vi "输入数据解析.vi"(0 "单个参数补充":dbl, 1 "从板号":dbl=1.0, 2 "主板二维码":string="BNET01", 3 "从板二维码":string="BNET01", 5 "主板引用":refnum<vi>, 7 "从板引用":refnum<vi>, 9 "主板选项":string="三级故障阀值", 11 "枚举":enum16{"主板", "从板"}(ring), 12 "快换":bool caption="快换写入") -> (4 "输出数组":dbl[][](array[numeric]), 6 "数组长度":dbl[](array[numeric]), 8 "循环次数":i32, 10 "命令":u32, 14 "名称":string[](array[string]), 15 "命令序号":u32[](array[numeric]))   [LabVIEW 2013] (continued)
                    n1944 = Unbundle By Name(w4966) -> ("总电压过低"=w4965:dbl)
                    n1945 = call "输入分辨率计算-EV05.vi"("1字节?"=FALSE, "数值"=w4965, "分辨率"=0.1) -> ("低字节"=w4968:dbl, "高字节1"=w4967:dbl)  [unwired: 2 in, 5 out]
                  }
                  frame Enabled {
                    w4971 = 255 ("高字节1")
                  }
                }
                n1946 = Build Array(w4963, w4964) -> (w4962:i32[])
              }
              frame 2 {
                # "温度过高"
                n1947 = disable-structure shown="启用" {
                  disable-tunnel: [w4978 255 ("高字节1")] -> w4974
                  disable-tunnel: w4972 -> [w4976 _]
                  frame Disabled {
                    n1948 = Unbundle By Name(w4976) -> ("温度过高"=w4975:dbl)
                    n1949 = call "输入分辨率计算-EV05.vi"("1字节?"=TRUE, "数值"=w4975, "偏移量"=-40.0, "分辨率"=1.0) -> ("高字节1"=w4978:dbl)  [unwired: 1 in, 6 out]
                  }
                  frame Enabled {
                  }
                }
                n1950 = Build Array(w4974) -> (w4973:i32[])
              }
              frame 3 {
                # "温度过低"
                n1951 = disable-structure shown="启用" {
                  disable-tunnel: [w4988 255 ("高字节1")] -> w4984
                  disable-tunnel: w4982 -> [w4986 _]
                  frame Disabled {
                    n1952 = Unbundle By Name(w4986) -> ("温度过低"=w4985:dbl)
                    n1953 = call "输入分辨率计算-EV05.vi"("1字节?"=TRUE, "数值"=w4985, "偏移量"=-40.0, "分辨率"=1.0) -> ("高字节1"=w4988:dbl)  [unwired: 1 in, 6 out]
                  }
                  frame Enabled {
                  }
                }
                n1954 = Build Array(w4984) -> (w4983:i32[])
              }
              frame 4 {
                # "整组温度不均衡"
                n1955 = disable-structure shown="启用" {
                  disable-tunnel: [w4998 255 ("高字节1")] -> w4994
                  disable-tunnel: w4992 -> [w4996 _]
                  frame Disabled {
                    n1956 = Unbundle By Name(w4996) -> ("整组温度不均衡"=w4995:dbl)
                    n1957 = call "输入分辨率计算-EV05.vi"("1字节?"=TRUE, "数值"=w4995, "偏移量"=0.0, "分辨率"=1.0) -> ("高字节1"=w4998:dbl)  [unwired: 1 in, 6 out]
                  }
                  frame Enabled {
                  }
                }
                n1958 = Build Array(w4994) -> (w4993:i32[])
              }
              frame 5 {
                # "单组电压不均衡"
                n1959 = disable-structure shown="启用" {
                  disable-tunnel: [w5010 w5013] -> w5005
                  disable-tunnel: [w5008 w5013] -> w5003
                  disable-tunnel: w5002 -> [w5007 _]
                  frame Enabled {
                    n1960 = Unbundle By Name(w5007) -> ("单组电压不均衡"=w5006:dbl)
                    n1961 = call "输入分辨率计算-EV05.vi"("1字节?"=FALSE, "数值"=w5006, "偏移量"=0.0, "分辨率"=0.001) -> ("低字节"=w5008:dbl, "高字节1"=w5010:dbl)  [unwired: 1 in, 5 out]
                  }
                  frame Disabled {
                    w5013 = 255 ("高字节1")
                  }
                }
                n1962 = Build Array(w5005, w5003) -> (w5004:dbl[])
              }
              frame 6 {
                # "整组电压不均衡"
                n1963 = disable-structure shown="启用" {
                  disable-tunnel: [w5022 w5025] -> w5017
                  disable-tunnel: [w5020 w5025] -> w5015
                  disable-tunnel: w5014 -> [w5019 _]
                  frame Disabled {
                    n1964 = Unbundle By Name(w5019) -> ("整组电压不均衡"=w5018:dbl)
                    n1965 = call "输入分辨率计算-EV05.vi"("1字节?"=FALSE, "数值"=w5018, "偏移量"=0.0, "分辨率"=0.001) -> ("低字节"=w5020:dbl, "高字节1"=w5022:dbl)  [unwired: 1 in, 5 out]
                  }
                  frame Enabled {
                    w5025 = 255 ("高字节1")
                  }
                }
                n1966 = Build Array(w5017, w5015) -> (w5016:i32[])
              }
              frame 7 {
                # "单体电压过高"
                n1967 = disable-structure shown="启用" {
                  disable-tunnel: [w5034 w5037] -> w5029
                  disable-tunnel: [w5032 w5037] -> w5027
                  disable-tunnel: w5026 -> [w5031 _]
                  frame Disabled {
                    n1968 = Unbundle By Name(w5031) -> ("单体电压过高"=w5030:dbl)
                    n1969 = call "输入分辨率计算-EV05.vi"("1字节?"=FALSE, "数值"=w5030, "偏移量"=0.0, "分辨率"=0.001) -> ("低字节"=w5032:dbl, "高字节1"=w5034:dbl)  [unwired: 1 in, 5 out]
                  }
                  frame Enabled {
                    w5037 = 255 ("高字节1")
                  }
                }
                n1970 = Build Array(w5029, w5027) -> (w5028:i32[])
              }
              frame 8 {
                # "单体电压过低"
                n1971 = disable-structure shown="启用" {
                  disable-tunnel: [w5046 w5049] -> w5041
                  disable-tunnel: [w5044 w5049] -> w5039
                  disable-tunnel: w5038 -> [w5043 _]
                  frame Disabled {
                    n1972 = Unbundle By Name(w5043) -> ("单体电压过低"=w5042:dbl)
                    n1973 = call "输入分辨率计算-EV05.vi"("1字节?"=FALSE, "数值"=w5042, "偏移量"=0.0, "分辨率"=0.001) -> ("低字节"=w5044:dbl, "高字节1"=w5046:dbl)  [unwired: 1 in, 5 out]
                  }
                  frame Enabled {
                    w5049 = 255 ("高字节1")
                  }
                }
                n1974 = Build Array(w5041, w5039) -> (w5040:i32[])
              }
              frame 9 {
                # "充电电流过高"
                n1975 = disable-structure shown="启用" {
                  disable-tunnel: [w5058 w5061] -> w5053
                  disable-tunnel: [w5056 w5061] -> w5051
                  disable-tunnel: w5050 -> [w5055 _]
                  frame Disabled {
                    n1976 = Unbundle By Name(w5055) -> ("充电电流过高"=w5054:dbl)
                    n1977 = call "输入分辨率计算-EV05.vi"("1字节?"=FALSE, "数值"=w5054, "偏移量"=-3000.0, "分辨率"=0.1) -> ("低字节"=w5056:dbl, "高字节1"=w5058:dbl)  [unwired: 1 in, 5 out]
                  }
                  frame Enabled {
                    w5061 = 255 ("高字节1")
                  }
                }
                n1978 = Build Array(w5053, w5051) -> (w5052:i32[])
              }
              frame 10 {
                # "放电电流过高"
                n1979 = disable-structure shown="启用" {
                  disable-tunnel: [w5070 w5073] -> w5065
                  disable-tunnel: [w5068 w5073] -> w5063
                  disable-tunnel: w5062 -> [w5067 _]
                  frame Disabled {
                    n1980 = Unbundle By Name(w5067) -> ("放电电流过高"=w5066:dbl)
                    n1981 = call "输入分辨率计算-EV05.vi"("1字节?"=FALSE, "数值"=w5066, "偏移量"=-3000.0, "分辨率"=0.1) -> ("低字节"=w5068:dbl, "高字节1"=w5070:dbl)  [unwired: 1 in, 5 out]
                  }
                  frame Enabled {
                    w5073 = 255 ("高字节1")
                  }
                }
                n1982 = Build Array(w5065, w5063) -> (w5064:i32[])
              }
              frame 11 {
                # "单组温度不均衡"
                n1983 = disable-structure shown="启用" {
                  disable-tunnel: [w5080 255 ("高字节1")] -> w5076
                  disable-tunnel: w5074 -> [w5078 _]
                  frame Disabled {
                    n1984 = Unbundle By Name(w5078) -> ("单组温度不均衡"=w5077:dbl)
                    n1985 = call "输入分辨率计算-EV05.vi"("1字节?"=TRUE, "数值"=w5077, "偏移量"=0.0, "分辨率"=1.0) -> ("高字节1"=w5080:dbl)  [unwired: 1 in, 6 out]
                  }
                  frame Enabled {
                  }
                }
                n1986 = Build Array(w5076) -> (w5075:i32[])
              }
              frame 12 {
                # "SOC过高"
                n1987 = Unbundle By Name(w5088) -> ("SOC过高"=w5087:dbl)
                n1988 = call "输入分辨率计算-EV05.vi"("1字节?"=FALSE, "数值"=w5087, "偏移量"=0.0, "分辨率"=0.1) -> ("低字节"=w5089:dbl, "高字节1"=w5090:dbl)  [unwired: 1 in, 5 out]
                n1989 = call "二进制解析-8.6.vi"("索引"=4, "数值"=w5090) -> ("低位子数组"=w5093:i32[])  [unwired: 3 out]
                n1990 = call "二进制解析-8.6.vi"("索引"=4, "数值"=w5089) -> ("低位子数组"=w5085:i32[], "高位子数组"=w5092:i32[])  [unwired: 2 out]
                n1991 = Insert Into Array(array=w5093, new element=w5092) -> (w5091:i32[])  [unwired: 1 in]
                n1992 = call "数值二进制转十进制-8.6.vi"("子数组"=w5091) -> ("十进制数值"=w5086:i32)  [unwired: 4 out]
                n1993 = disable-structure shown="启用" {
                  disable-tunnel: w5086 -> [w5101 _]
                  disable-tunnel: [w5101 255 ("高字节1")] -> w5084
                  disable-tunnel: [w5100 i32[] [] ("低位子数组 23")] -> _
                  disable-tunnel: w5085 -> [w5100 _]
                  frame Disabled {
                  }
                  frame Enabled {
                  }
                }
                n1994 = Build Array(w5084, w5084) -> (w5097:i32[])
              }
              frame 13 {
                # "SOC过低"
                n1995 = Unbundle By Name(w5110) -> ("SOC过低"=w5109:dbl)
                n1996 = call "输入分辨率计算-EV05.vi"("1字节?"=FALSE, "数值"=w5109, "偏移量"=0.0, "分辨率"=0.1) -> ("低字节"=w5107:dbl, "高字节1"=w5108:dbl)  [unwired: 1 in, 5 out]
                n1997 = call "二进制解析-8.6.vi"("索引"=4, "数值"=w5108) -> ("低位子数组"=w5105:i32[])  [unwired: 3 out]
                n1998 = disable-structure shown="启用" {
                  disable-tunnel: w5107 -> [w5117 _]
                  disable-tunnel: [w5117 255 ("高字节1")] -> w5106
                  disable-tunnel: w5105 -> [w5116 _]
                  disable-tunnel: [_ 255 ("高字节1")] -> w5104
                  frame Disabled {
                    (unwired) i32[] [] ("低位子数组 4")
                  }
                  frame Enabled {
                  }
                }
                n1999 = Build Array(w5104, w5106) -> (w5113:i32[])
              }
              frame 14 {
                # "内阻过大"
                n2000 = disable-structure shown="启用" {
                  disable-tunnel: w5122 -> [w5127 _]
                  disable-tunnel: [w5123 255 ("高字节1")] -> w5120
                  frame Disabled {
                    n2001 = Unbundle By Name(w5127) -> ("内阻过大"=w5126:dbl)
                    n2002 = call "输入分辨率计算-EV05.vi"("1字节?"=TRUE, "数值"=w5126, "分辨率"=0.1) -> ("高字节1"=w5123:dbl)  [unwired: 2 in, 6 out]
                  }
                  frame Enabled {
                  }
                }
                n2003 = Build Array(w5120) -> (w5121:i32[])
              }
              frame 15 {
                # "极柱温度过高"
                n2004 = disable-structure shown="启用" {
                  disable-tunnel: w5131 -> [w5137 _]
                  disable-tunnel: [w5133 255 ("高字节1")] -> w5129
                  frame Disabled {
                    n2005 = Unbundle By Name(w5137) -> ("极柱温度过高"=w5136:dbl)
                    n2006 = call "输入分辨率计算-EV05.vi"("1字节?"=TRUE, "数值"=w5136, "偏移量"=-40.0, "分辨率"=1.0) -> ("高字节1"=w5133:dbl)  [unwired: 1 in, 6 out]
                  }
                  frame Enabled {
                  }
                }
                n2007 = Build Array(w5129) -> (w5130:i32[])
              }
              frame 16 {
                # "SOH过低"
                n2008 = disable-structure shown="启用" {
                  disable-tunnel: [w5154 w5162] -> w5141
                  disable-tunnel: w5140 -> [w5151 _]
                  disable-tunnel: [w5143 w5162] -> w5139
                  frame Disabled {
                    n2009 = Unbundle By Name(w5151) -> ("SOH过低"=w5150:dbl)
                    n2010 = call "输入分辨率计算-EV05.vi"("1字节?"=FALSE, "数值"=w5150, "偏移量"=0.0, "分辨率"=0.1) -> ("低字节"=w5152:dbl, "高字节1"=w5153:dbl)  [unwired: 1 in, 5 out]
                    n2011 = call "二进制解析-8.6.vi"("索引"=4, "数值"=w5153) -> ("低位子数组"=w5156:i32[])  [unwired: 3 out]
                    n2012 = call "二进制解析-8.6.vi"("索引"=4, "数值"=w5152) -> ("低位子数组"=w5145:i32[], "高位子数组"=w5155:i32[])  [unwired: 2 out]
                    n2013 = call "二进制解析-8.6.vi"("索引"=4, "数值"=0) -> ("低位子数组"=w5146:i32[])  [unwired: 3 out]
                    n2014 = Insert Into Array(array=w5156, new element=w5155) -> (w5149:i32[])  [unwired: 1 in]
                    n2015 = Insert Into Array(array=w5145, new element=w5146) -> (w5144:i32[])  [unwired: 1 in]
                    n2016 = call "数值二进制转十进制-8.6.vi"("子数组"=w5149) -> ("十进制数值"=w5154:i32)  [unwired: 4 out]
                    n2017 = call "数值二进制转十进制-8.6.vi"("子数组"=w5144) -> ("十进制数值"=w5143:i32)  [unwired: 4 out]
                  }
                  frame Enabled {
                    w5162 = 255 ("高字节1")
                  }
                }
                n2018 = Build Array(w5141, w5139) -> (w5142:i32[])
              }
            }
            n2019 = Insert Into Array(array=w4946, new element=w4947) -> (w4945:dbl[])  [unwired: 1 in]
          }
          n2020 = Build Array(w4942) -> (w4941:dbl[][])
          n2021 = Build Array("三级故障阀值") -> (w4932:string[])
        }
        frame "整组电压不均衡" {
          n2022 = Unbundle By Name(w5168) -> ("一级故障"=w5169:refnum<vi>)
          n2023 = property class="Clust (严格)"(reference=w5169) -> ("Value"=w5167:T4)  [unwired: 1 in, 2 out]
          n2024 = for {
            N: 17 -> [_]
            tunnel: w5167 -> [w5179]
            shift-right: [w5176] -> w5173
            shift-left: dbl[] [] -> [w5177]
            i -> [w5180]
            n2025 = case shown="13" w5180 {
              tunnel: w5179 -> [w5181 w5192 w5203 w5213 w5223 w5233 w5245 w5257 w5269 w5281 w5293 w5305 w5319 w5340 w5351 w5360 w5369]
              tunnel: [w5182 w5193 w5204 w5214 w5224 w5235 w5247 w5259 w5271 w5283 w5295 w5306 w5328 w5343 w5350 w5359 w5371] -> w5178
              frame 0, Default {
                # "总电压过高"
                n2026 = disable-structure shown="启用" {
                  disable-tunnel: [w5188 w5191] -> w5184
                  disable-tunnel: [w5187 w5191] -> w5183
                  disable-tunnel: w5181 -> [w5186 _]
                  frame Disabled {
                    n2027 = Unbundle By Name(w5186) -> ("总电压过高"=w5185:dbl)
                    n2028 = call "输入分辨率计算-EV05.vi"("1字节?"=FALSE, "数值"=w5185, "分辨率"=0.1) -> ("低字节"=w5188:dbl, "高字节1"=w5187:dbl)  [unwired: 2 in, 5 out]
                  }
                  frame Enabled {
                    w5191 = 255 ("高字节1")
                  }
                }
                n2029 = Build Array(w5183, w5184) -> (w5182:i32[])
              }
              frame 1 {
                # "总电压过低"
                n2030 = disable-structure shown="启用" {
                  disable-tunnel: [w5199 w5202] -> w5195
                  disable-tunnel: [w5198 w5202] -> w5194
                  disable-tunnel: w5192 -> [w5197 _]
                  frame Disabled {
                    n2031 = Unbundle By Name(w5197) -> ("总电压过低"=w5196:dbl)
                    n2032 = call "输入分辨率计算-EV05.vi"("1字节?"=FALSE, "数值"=w5196, "分辨率"=0.1) -> ("低字节"=w5199:dbl, "高字节1"=w5198:dbl)  [unwired: 2 in, 5 out]
                  }
                  frame Enabled {
                    w5202 = 255 ("高字节1")
                  }
                }
                n2033 = Build Array(w5194, w5195) -> (w5193:i32[])
              }
              frame 2 {
                # "温度过高"
                n2034 = disable-structure shown="启用" {
                  disable-tunnel: [w5209 255 ("高字节1")] -> w5205
                  disable-tunnel: w5203 -> [w5207 _]
                  frame Disabled {
                    n2035 = Unbundle By Name(w5207) -> ("温度过高"=w5206:dbl)
                    n2036 = call "输入分辨率计算-EV05.vi"("1字节?"=TRUE, "数值"=w5206, "偏移量"=-40.0, "分辨率"=1.0) -> ("高字节1"=w5209:dbl)  [unwired: 1 in, 6 out]
                  }
                  frame Enabled {
                  }
                }
                n2037 = Build Array(w5205) -> (w5204:i32[])
              }
              frame 3 {
                # "温度过低"
                n2038 = disable-structure shown="启用" {
                  disable-tunnel: [w5219 255 ("高字节1")] -> w5215
                  disable-tunnel: w5213 -> [w5217 _]
                  frame Disabled {
                    n2039 = Unbundle By Name(w5217) -> ("温度过低"=w5216:dbl)
                    n2040 = call "输入分辨率计算-EV05.vi"("1字节?"=TRUE, "数值"=w5216, "偏移量"=-40.0, "分辨率"=1.0) -> ("高字节1"=w5219:dbl)  [unwired: 1 in, 6 out]
                  }
                  frame Enabled {
                  }
                }
                n2041 = Build Array(w5215) -> (w5214:i32[])
              }
              frame 4 {
                # "整组温度不均衡"
                n2042 = disable-structure shown="启用" {
                  disable-tunnel: [w5229 255 ("高字节1")] -> w5225
                  disable-tunnel: w5223 -> [w5227 _]
                  frame Disabled {
                    n2043 = Unbundle By Name(w5227) -> ("整组温度不均衡"=w5226:dbl)
                    n2044 = call "输入分辨率计算-EV05.vi"("1字节?"=TRUE, "数值"=w5226, "偏移量"=0.0, "分辨率"=1.0) -> ("高字节1"=w5229:dbl)  [unwired: 1 in, 6 out]
                  }
                  frame Enabled {
                  }
                }
                n2045 = Build Array(w5225) -> (w5224:i32[])
              }
              frame 5 {
                # "单组电压不均衡"
                n2046 = disable-structure shown="启用" {
                  disable-tunnel: [w5241 w5244] -> w5236
                  disable-tunnel: [w5239 w5244] -> w5234
                  disable-tunnel: w5233 -> [w5238 _]
                  frame Disabled {
                    n2047 = Unbundle By Name(w5238) -> ("单组电压不均衡"=w5237:dbl)
                    n2048 = call "输入分辨率计算-EV05.vi"("1字节?"=FALSE, "数值"=w5237, "偏移量"=0.0, "分辨率"=0.001) -> ("低字节"=w5239:dbl, "高字节1"=w5241:dbl)  [unwired: 1 in, 5 out]
                  }
                  frame Enabled {
                    w5244 = 255 ("高字节1")
                  }
                }
                n2049 = Build Array(w5236, w5234) -> (w5235:i32[])
              }
              frame 6 {
                # "整组电压不均衡"
                n2050 = disable-structure shown="启用" {
                  disable-tunnel: [w5253 w5256] -> w5248
                  disable-tunnel: [w5251 w5256] -> w5246
                  disable-tunnel: w5245 -> [w5250 _]
                  frame Enabled {
                    n2051 = Unbundle By Name(w5250) -> ("整组电压不均衡"=w5249:dbl)
                    n2052 = call "输入分辨率计算-EV05.vi"("1字节?"=FALSE, "数值"=w5249, "偏移量"=0.0, "分辨率"=0.001) -> ("低字节"=w5251:dbl, "高字节1"=w5253:dbl)  [unwired: 1 in, 5 out]
                  }
                  frame Disabled {
                    w5256 = 255 ("高字节1")
                  }
                }
                n2053 = Build Array(w5248, w5246) -> (w5247:dbl[])
              }
              frame 7 {
                # "单体电压过高"
                n2054 = disable-structure shown="启用" {
                  disable-tunnel: [w5265 w5268] -> w5260
                  disable-tunnel: [w5263 w5268] -> w5258
                  disable-tunnel: w5257 -> [w5262 _]
                  frame Disabled {
                    n2055 = Unbundle By Name(w5262) -> ("单体电压过高"=w5261:dbl)
                    n2056 = call "输入分辨率计算-EV05.vi"("1字节?"=FALSE, "数值"=w5261, "偏移量"=0.0, "分辨率"=0.001) -> ("低字节"=w5263:dbl, "高字节1"=w5265:dbl)  [unwired: 1 in, 5 out]
                  }
                  frame Enabled {
                    w5268 = 255 ("高字节1")
                  }
                }
                n2057 = Build Array(w5260, w5258) -> (w5259:i32[])
              }
              frame 8 {
                # "单体电压过低"
                n2058 = disable-structure shown="启用" {
                  disable-tunnel: [w5277 w5280] -> w5272
                  disable-tunnel: [w5275 w5280] -> w5270
                  disable-tunnel: w5269 -> [w5274 _]
                  frame Disabled {
                    n2059 = Unbundle By Name(w5274) -> ("单体电压过低"=w5273:dbl)
                    n2060 = call "输入分辨率计算-EV05.vi"("1字节?"=FALSE, "数值"=w5273, "偏移量"=0.0, "分辨率"=0.001) -> ("低字节"=w5275:dbl, "高字节1"=w5277:dbl)  [unwired: 1 in, 5 out]
                  }
                  frame Enabled {
                    w5280 = 255 ("高字节1")
                  }
                }
                n2061 = Build Array(w5272, w5270) -> (w5271:i32[])
              }
              frame 9 {
                # "充电电流过高"
                n2062 = disable-structure shown="启用" {
                  disable-tunnel: [w5289 w5292] -> w5284
                  disable-tunnel: [w5287 w5292] -> w5282
                  disable-tunnel: w5281 -> [w5286 _]
                  frame Disabled {
                    n2063 = Unbundle By Name(w5286) -> ("充电电流过高"=w5285:dbl)
                    n2064 = call "输入分辨率计算-EV05.vi"("1字节?"=FALSE, "数值"=w5285, "偏移量"=-3000.0, "分辨率"=0.1) -> ("低字节"=w5287:dbl, "高字节1"=w5289:dbl)  [unwired: 1 in, 5 out]
                  }
                  frame Enabled {
                    w5292 = 255 ("高字节1")
                  }
                }
                n2065 = Build Array(w5284, w5282) -> (w5283:i32[])
              }
              frame 10 {
                # "放电电流过高"
                n2066 = disable-structure shown="启用" {
                  disable-tunnel: [w5301 w5304] -> w5296
                  disable-tunnel: [w5299 w5304] -> w5294
                  disable-tunnel: w5293 -> [w5298 _]
                  frame Disabled {
                    n2067 = Unbundle By Name(w5298) -> ("放电电流过高"=w5297:dbl)
                    n2068 = call "输入分辨率计算-EV05.vi"("1字节?"=FALSE, "数值"=w5297, "偏移量"=-3000.0, "分辨率"=0.1) -> ("低字节"=w5299:dbl, "高字节1"=w5301:dbl)  [unwired: 1 in, 5 out]
                  }
                  frame Enabled {
                    w5304 = 255 ("高字节1")
                  }
                }
                n2069 = Build Array(w5296, w5294) -> (w5295:i32[])
              }
              frame 11 {
                # "单组温度不均衡"
                n2070 = disable-structure shown="启用" {
                  disable-tunnel: [w5311 255 ("高字节1")] -> w5307
                  disable-tunnel: w5305 -> [w5309 _]
                  frame Disabled {
                    n2071 = Unbundle By Name(w5309) -> ("单组温度不均衡"=w5308:dbl)
                    n2072 = call "输入分辨率计算-EV05.vi"("1字节?"=TRUE, "数值"=w5308, "偏移量"=0.0, "分辨率"=1.0) -> ("高字节1"=w5311:dbl)  [unwired: 1 in, 6 out]
                  }
                  frame Enabled {
                  }
                }
                n2073 = Build Array(w5307) -> (w5306:i32[])
              }
              frame 12 {
                # "SOC过高"
                n2074 = Unbundle By Name(w5319) -> ("SOC过高"=w5318:dbl)
                n2075 = call "输入分辨率计算-EV05.vi"("1字节?"=FALSE, "数值"=w5318, "偏移量"=0.0, "分辨率"=0.1) -> ("低字节"=w5320:dbl, "高字节1"=w5321:dbl)  [unwired: 1 in, 5 out]
                n2076 = call "二进制解析-8.6.vi"("索引"=4, "数值"=w5321) -> ("低位子数组"=w5324:i32[])  [unwired: 3 out]
                n2077 = call "二进制解析-8.6.vi"("索引"=4, "数值"=w5320) -> ("低位子数组"=w5316:i32[], "高位子数组"=w5323:i32[])  [unwired: 2 out]
                n2078 = Insert Into Array(array=w5324, new element=w5323) -> (w5322:i32[])  [unwired: 1 in]
                n2079 = call "数值二进制转十进制-8.6.vi"("子数组"=w5322) -> ("十进制数值"=w5317:i32)  [unwired: 4 out]
                n2080 = disable-structure shown="启用" {
                  disable-tunnel: w5317 -> [w5332 _]
                  disable-tunnel: [w5332 255 ("高字节1")] -> w5315
                  disable-tunnel: [w5331 i32[] [] ("低位子数组 24")] -> _
                  disable-tunnel: w5316 -> [w5331 _]
                  frame Disabled {
                  }
                  frame Enabled {
                  }
                }
                n2081 = Build Array(w5315, w5315) -> (w5328:i32[])
              }
              frame 13 {
                # "SOC过低"
                n2082 = Unbundle By Name(w5340) -> ("SOC过低"=w5339:dbl)
                n2083 = call "输入分辨率计算-EV05.vi"("1字节?"=FALSE, "数值"=w5339, "偏移量"=0.0, "分辨率"=0.1) -> ("低字节"=w5337:dbl, "高字节1"=w5338:dbl)  [unwired: 1 in, 5 out]
                n2084 = call "二进制解析-8.6.vi"("索引"=4, "数值"=w5338) -> ("低位子数组"=w5336:i32[])  [unwired: 3 out]
                n2085 = disable-structure shown="启用" {
                  disable-tunnel: w5337 -> [w5347 _]
                  disable-tunnel: [w5347 255 ("高字节1")] -> w5335
                  disable-tunnel: w5336 -> [w5346 _]
                  frame Disabled {
                    (unwired) i32[] [] ("低位子数组 4")
                  }
                  frame Enabled {
                  }
                }
                n2086 = Build Array(w5335, w5335) -> (w5343:i32[])
              }
              frame 14 {
                # "内阻过大"
                n2087 = disable-structure shown="启用" {
                  disable-tunnel: w5351 -> [w5356 _]
                  disable-tunnel: [w5352 255 ("高字节1")] -> w5349
                  frame Disabled {
                    n2088 = Unbundle By Name(w5356) -> ("内阻过大"=w5355:dbl)
                    n2089 = call "输入分辨率计算-EV05.vi"("1字节?"=TRUE, "数值"=w5355, "分辨率"=0.1) -> ("高字节1"=w5352:dbl)  [unwired: 2 in, 6 out]
                  }
                  frame Enabled {
                  }
                }
                n2090 = Build Array(w5349) -> (w5350:i32[])
              }
              frame 15 {
                # "极柱温度过高"
                n2091 = disable-structure shown="启用" {
                  disable-tunnel: w5360 -> [w5366 _]
                  disable-tunnel: [w5362 255 ("高字节1")] -> w5358
                  frame Disabled {
                    n2092 = Unbundle By Name(w5366) -> ("极柱温度过高"=w5365:dbl)
                    n2093 = call "输入分辨率计算-EV05.vi"("1字节?"=TRUE, "数值"=w5365, "偏移量"=-40.0, "分辨率"=1.0) -> ("高字节1"=w5362:dbl)  [unwired: 1 in, 6 out]
                  }
                  frame Enabled {
                  }
                }
                n2094 = Build Array(w5358) -> (w5359:i32[])
              }
              frame 16 {
                # "SOH过低"
                n2095 = disable-structure shown="启用" {
                  disable-tunnel: [w5383 w5391] -> w5370
                  disable-tunnel: w5369 -> [w5380 _]
                  disable-tunnel: [w5372 w5391] -> w5368
                  frame Disabled {
                    n2096 = Unbundle By Name(w5380) -> ("SOH过低"=w5379:dbl)
                    n2097 = call "输入分辨率计算-EV05.vi"("1字节?"=FALSE, "数值"=w5379, "偏移量"=0.0, "分辨率"=0.1) -> ("低字节"=w5381:dbl, "高字节1"=w5382:dbl)  [unwired: 1 in, 5 out]
                    n2098 = call "二进制解析-8.6.vi"("索引"=4, "数值"=w5382) -> ("低位子数组"=w5385:i32[])  [unwired: 3 out]
                    n2099 = call "二进制解析-8.6.vi"("索引"=4, "数值"=w5381) -> ("低位子数组"=w5374:i32[], "高位子数组"=w5384:i32[])  [unwired: 2 out]
                    n2100 = call "二进制解析-8.6.vi"("索引"=4, "数值"=0) -> ("低位子数组"=w5375:i32[])  [unwired: 3 out]
                    n2101 = Insert Into Array(array=w5385, new element=w5384) -> (w5378:i32[])  [unwired: 1 in]
                    n2102 = Insert Into Array(array=w5374, new element=w5375) -> (w5373:i32[])  [unwired: 1 in]
                    n2103 = call "数值二进制转十进制-8.6.vi"("子数组"=w5378) -> ("十进制数值"=w5383:i32)  [unwired: 4 out]
                    n2104 = call "数值二进制转十进制-8.6.vi"("子数组"=w5373) -> ("十进制数值"=w5372:i32)  [unwired: 4 out]
                  }
                  frame Enabled {
                    w5391 = 255 ("高字节1")
                  }
                }
                n2105 = Build Array(w5370, w5368) -> (w5371:i32[])
              }
            }
            n2106 = Insert Into Array(array=w5177, new element=w5178) -> (w5176:dbl[])  [unwired: 1 in]
          }
          n2107 = Build Array(w5173) -> (w5172:dbl[][])
          n2108 = Build Array("一级故障阀值") -> (w5163:string[])
        }
        frame "整组电压不均衡(2)" {
          n2109 = Unbundle By Name(w5397) -> ("一级故障 2"=w5398:refnum<vi>)
          n2110 = property class="Clust (严格)"(reference=w5398) -> ("Value"=w5396:T4)  [unwired: 1 in, 2 out]
          n2111 = for {
            N: 17 -> [_]
            tunnel: w5396 -> [w5408]
            shift-right: [w5405] -> w5402
            shift-left: dbl[] [] -> [w5406]
            i -> [w5409]
            n2112 = case shown="13" w5409 {
              tunnel: w5408 -> [w5410 w5421 w5432 w5442 w5452 w5462 w5474 w5486 w5498 w5510 w5522 w5534 w5548 w5569 w5580 w5589 w5598]
              tunnel: [w5411 w5422 w5433 w5443 w5453 w5464 w5476 w5488 w5500 w5512 w5524 w5535 w5557 w5572 w5579 w5588 w5600] -> w5407
              frame 0, Default {
                # "总电压过高"
                n2113 = disable-structure shown="启用" {
                  disable-tunnel: [w5417 w5420] -> w5413
                  disable-tunnel: [w5416 w5420] -> w5412
                  disable-tunnel: w5410 -> [w5415 _]
                  frame Disabled {
                    n2114 = Unbundle By Name(w5415) -> ("总电压过高"=w5414:dbl)
                    n2115 = call "输入分辨率计算-EV05.vi"("1字节?"=FALSE, "数值"=w5414, "分辨率"=0.1) -> ("低字节"=w5417:dbl, "高字节1"=w5416:dbl)  [unwired: 2 in, 5 out]
                  }
                  frame Enabled {
                    w5420 = 255 ("高字节1")
                  }
                }
                n2116 = Build Array(w5412, w5413) -> (w5411:i32[])
              }
              frame 1 {
                # "总电压过低"
                n2117 = disable-structure shown="启用" {
                  disable-tunnel: [w5428 w5431] -> w5424
                  disable-tunnel: [w5427 w5431] -> w5423
                  disable-tunnel: w5421 -> [w5426 _]
                  frame Disabled {
                    n2118 = Unbundle By Name(w5426) -> ("总电压过低"=w5425:dbl)
                    n2119 = call "输入分辨率计算-EV05.vi"("1字节?"=FALSE, "数值"=w5425, "分辨率"=0.1) -> ("低字节"=w5428:dbl, "高字节1"=w5427:dbl)  [unwired: 2 in, 5 out]
                  }
                  frame Enabled {
                    w5431 = 255 ("高字节1")
                  }
                }
                n2120 = Build Array(w5423, w5424) -> (w5422:i32[])
              }
              frame 2 {
                # "温度过高"
                n2121 = disable-structure shown="启用" {
                  disable-tunnel: [w5438 255 ("高字节1")] -> w5434
                  disable-tunnel: w5432 -> [w5436 _]
                  frame Disabled {
                    n2122 = Unbundle By Name(w5436) -> ("温度过高"=w5435:dbl)
                    n2123 = call "输入分辨率计算-EV05.vi"("1字节?"=TRUE, "数值"=w5435, "偏移量"=-40.0, "分辨率"=1.0) -> ("高字节1"=w5438:dbl)  [unwired: 1 in, 6 out]
                  }
                  frame Enabled {
                  }
                }
                n2124 = Build Array(w5434) -> (w5433:i32[])
              }
              frame 3 {
                # "温度过低"
                n2125 = disable-structure shown="启用" {
                  disable-tunnel: [w5448 255 ("高字节1")] -> w5444
                  disable-tunnel: w5442 -> [w5446 _]
                  frame Disabled {
                    n2126 = Unbundle By Name(w5446) -> ("温度过低"=w5445:dbl)
                    n2127 = call "输入分辨率计算-EV05.vi"("1字节?"=TRUE, "数值"=w5445, "偏移量"=-40.0, "分辨率"=1.0) -> ("高字节1"=w5448:dbl)  [unwired: 1 in, 6 out]
                  }
                  frame Enabled {
                  }
                }
                n2128 = Build Array(w5444) -> (w5443:i32[])
              }
              frame 4 {
                # "整组温度不均衡"
                n2129 = disable-structure shown="启用" {
                  disable-tunnel: [w5458 255 ("高字节1")] -> w5454
                  disable-tunnel: w5452 -> [w5456 _]
                  frame Disabled {
                    n2130 = Unbundle By Name(w5456) -> ("整组温度不均衡"=w5455:dbl)
                    n2131 = call "输入分辨率计算-EV05.vi"("1字节?"=TRUE, "数值"=w5455, "偏移量"=0.0, "分辨率"=1.0) -> ("高字节1"=w5458:dbl)  [unwired: 1 in, 6 out]
                  }
                  frame Enabled {
                  }
                }
                n2132 = Build Array(w5454) -> (w5453:i32[])
              }
              frame 5 {
                # "单组电压不均衡"
                n2133 = disable-structure shown="启用" {
                  disable-tunnel: [w5470 w5473] -> w5465
                  disable-tunnel: [w5468 w5473] -> w5463
                  disable-tunnel: w5462 -> [w5467 _]
                  frame Disabled {
                    n2134 = Unbundle By Name(w5467) -> ("单组电压不均衡"=w5466:dbl)
                    n2135 = call "输入分辨率计算-EV05.vi"("1字节?"=FALSE, "数值"=w5466, "偏移量"=0.0, "分辨率"=0.001) -> ("低字节"=w5468:dbl, "高字节1"=w5470:dbl)  [unwired: 1 in, 5 out]
                  }
                  frame Enabled {
                    w5473 = 255 ("高字节1")
                  }
                }
                n2136 = Build Array(w5465, w5463) -> (w5464:i32[])
              }
              frame 6 {
                # "整组电压不均衡"
                n2137 = disable-structure shown="启用" {
                  disable-tunnel: [w5482 w5485] -> w5477
                  disable-tunnel: [w5480 w5485] -> w5475
                  disable-tunnel: w5474 -> [w5479 _]
                  frame Enabled {
                    n2138 = Unbundle By Name(w5479) -> ("整组电压不均衡"=w5478:dbl)
                    n2139 = call "输入分辨率计算-EV05.vi"("1字节?"=FALSE, "数值"=w5478, "偏移量"=0.0, "分辨率"=0.001) -> ("低字节"=w5480:dbl, "高字节1"=w5482:dbl)  [unwired: 1 in, 5 out]
                  }
                  frame Disabled {
                    w5485 = 255 ("高字节1")
                  }
                }
                n2140 = Build Array(w5477, w5475) -> (w5476:dbl[])
              }
              frame 7 {
                # "单体电压过高"
                n2141 = disable-structure shown="启用" {
                  disable-tunnel: [w5494 w5497] -> w5489
                  disable-tunnel: [w5492 w5497] -> w5487
                  disable-tunnel: w5486 -> [w5491 _]
                  frame Disabled {
                    n2142 = Unbundle By Name(w5491) -> ("单体电压过高"=w5490:dbl)
                    n2143 = call "输入分辨率计算-EV05.vi"("1字节?"=FALSE, "数值"=w5490, "偏移量"=0.0, "分辨率"=0.001) -> ("低字节"=w5492:dbl, "高字节1"=w5494:dbl)  [unwired: 1 in, 5 out]
                  }
                  frame Enabled {
                    w5497 = 255 ("高字节1")
                  }
                }
                n2144 = Build Array(w5489, w5487) -> (w5488:i32[])
              }
              frame 8 {
                # "单体电压过低"
                n2145 = disable-structure shown="启用" {
                  disable-tunnel: [w5506 w5509] -> w5501
                  disable-tunnel: [w5504 w5509] -> w5499
                  disable-tunnel: w5498 -> [w5503 _]
                  frame Disabled {
                    n2146 = Unbundle By Name(w5503) -> ("单体电压过低"=w5502:dbl)
                    n2147 = call "输入分辨率计算-EV05.vi"("1字节?"=FALSE, "数值"=w5502, "偏移量"=0.0, "分辨率"=0.001) -> ("低字节"=w5504:dbl, "高字节1"=w5506:dbl)  [unwired: 1 in, 5 out]
                  }
                  frame Enabled {
                    w5509 = 255 ("高字节1")
                  }
                }
                n2148 = Build Array(w5501, w5499) -> (w5500:i32[])
              }
              frame 9 {
                # "充电电流过高"
                n2149 = disable-structure shown="启用" {
                  disable-tunnel: [w5518 w5521] -> w5513
                  disable-tunnel: [w5516 w5521] -> w5511
                  disable-tunnel: w5510 -> [w5515 _]
                  frame Disabled {
                    n2150 = Unbundle By Name(w5515) -> ("充电电流过高"=w5514:dbl)
                    n2151 = call "输入分辨率计算-EV05.vi"("1字节?"=FALSE, "数值"=w5514, "偏移量"=-3000.0, "分辨率"=0.1) -> ("低字节"=w5516:dbl, "高字节1"=w5518:dbl)  [unwired: 1 in, 5 out]
                  }
                  frame Enabled {
                    w5521 = 255 ("高字节1")
                  }
                }
                n2152 = Build Array(w5513, w5511) -> (w5512:i32[])
              }
              frame 10 {
                # "放电电流过高"
                n2153 = disable-structure shown="启用" {
                  disable-tunnel: [w5530 w5533] -> w5525
                  disable-tunnel: [w5528 w5533] -> w5523
                  disable-tunnel: w5522 -> [w5527 _]
                  frame Disabled {
                    n2154 = Unbundle By Name(w5527) -> ("放电电流过高"=w5526:dbl)
                    n2155 = call "输入分辨率计算-EV05.vi"("1字节?"=FALSE, "数值"=w5526, "偏移量"=-3000.0, "分辨率"=0.1) -> ("低字节"=w5528:dbl, "高字节1"=w5530:dbl)  [unwired: 1 in, 5 out]
                  }
                  frame Enabled {
                    w5533 = 255 ("高字节1")
                  }
                }
                n2156 = Build Array(w5525, w5523) -> (w5524:i32[])
              }
              frame 11 {
                # "单组温度不均衡"
                n2157 = disable-structure shown="启用" {
                  disable-tunnel: [w5540 255 ("高字节1")] -> w5536
                  disable-tunnel: w5534 -> [w5538 _]
                  frame Disabled {
                    n2158 = Unbundle By Name(w5538) -> ("单组温度不均衡"=w5537:dbl)
                    n2159 = call "输入分辨率计算-EV05.vi"("1字节?"=TRUE, "数值"=w5537, "偏移量"=0.0, "分辨率"=1.0) -> ("高字节1"=w5540:dbl)  [unwired: 1 in, 6 out]
                  }
                  frame Enabled {
                  }
                }
                n2160 = Build Array(w5536) -> (w5535:i32[])
              }
              frame 12 {
                # "SOC过高"
                n2161 = Unbundle By Name(w5548) -> ("SOC过高"=w5547:dbl)
                n2162 = call "输入分辨率计算-EV05.vi"("1字节?"=FALSE, "数值"=w5547, "偏移量"=0.0, "分辨率"=0.1) -> ("低字节"=w5549:dbl, "高字节1"=w5550:dbl)  [unwired: 1 in, 5 out]
                n2163 = call "二进制解析-8.6.vi"("索引"=4, "数值"=w5550) -> ("低位子数组"=w5553:i32[])  [unwired: 3 out]
                n2164 = call "二进制解析-8.6.vi"("索引"=4, "数值"=w5549) -> ("低位子数组"=w5545:i32[], "高位子数组"=w5552:i32[])  [unwired: 2 out]
                n2165 = Insert Into Array(array=w5553, new element=w5552) -> (w5551:i32[])  [unwired: 1 in]
                n2166 = call "数值二进制转十进制-8.6.vi"("子数组"=w5551) -> ("十进制数值"=w5546:i32)  [unwired: 4 out]
                n2167 = disable-structure shown="启用" {
                  disable-tunnel: w5546 -> [w5561 _]
                  disable-tunnel: [w5561 255 ("高字节1")] -> w5544
                  disable-tunnel: [w5560 i32[] [] ("低位子数组 24")] -> _
                  disable-tunnel: w5545 -> [w5560 _]
                  frame Disabled {
                  }
                  frame Enabled {
                  }
                }
                n2168 = Build Array(w5544, w5544) -> (w5557:i32[])
              }
              frame 13 {
                # "SOC过低"
                n2169 = Unbundle By Name(w5569) -> ("SOC过低"=w5568:dbl)
                n2170 = call "输入分辨率计算-EV05.vi"("1字节?"=FALSE, "数值"=w5568, "偏移量"=0.0, "分辨率"=0.1) -> ("低字节"=w5566:dbl, "高字节1"=w5567:dbl)  [unwired: 1 in, 5 out]
                n2171 = call "二进制解析-8.6.vi"("索引"=4, "数值"=w5567) -> ("低位子数组"=w5565:i32[])  [unwired: 3 out]
                n2172 = disable-structure shown="启用" {
                  disable-tunnel: w5566 -> [w5576 _]
                  disable-tunnel: [w5576 255 ("高字节1")] -> w5564
                  disable-tunnel: w5565 -> [w5575 _]
                  frame Disabled {
                    (unwired) i32[] [] ("低位子数组 4")
                  }
                  frame Enabled {
                  }
                }
                n2173 = Build Array(w5564, w5564) -> (w5572:i32[])
              }
              frame 14 {
                # "内阻过大"
                n2174 = disable-structure shown="启用" {
                  disable-tunnel: w5580 -> [w5585 _]
                  disable-tunnel: [w5581 255 ("高字节1")] -> w5578
                  frame Disabled {
                    n2175 = Unbundle By Name(w5585) -> ("内阻过大"=w5584:dbl)
                    n2176 = call "输入分辨率计算-EV05.vi"("1字节?"=TRUE, "数值"=w5584, "分辨率"=0.1) -> ("高字节1"=w5581:dbl)  [unwired: 2 in, 6 out]
                  }
                  frame Enabled {
                  }
                }
                n2177 = Build Array(w5578) -> (w5579:i32[])
              }
              frame 15 {
                # "极柱温度过高"
                n2178 = disable-structure shown="启用" {
                  disable-tunnel: w5589 -> [w5595 _]
                  disable-tunnel: [w5591 255 ("高字节1")] -> w5587
                  frame Disabled {
                    n2179 = Unbundle By Name(w5595) -> ("极柱温度过高"=w5594:dbl)
                    n2180 = call "输入分辨率计算-EV05.vi"("1字节?"=TRUE, "数值"=w5594, "偏移量"=-40.0, "分辨率"=1.0) -> ("高字节1"=w5591:dbl)  [unwired: 1 in, 6 out]
                  }
                  frame Enabled {
                  }
                }
                n2181 = Build Array(w5587) -> (w5588:i32[])
              }
              frame 16 {
                # "SOH过低"
                n2182 = disable-structure shown="启用" {
                  disable-tunnel: [w5612 w5620] -> w5599
                  disable-tunnel: w5598 -> [w5609 _]
                  disable-tunnel: [w5601 w5620] -> w5597
                  frame Disabled {
                    n2183 = Unbundle By Name(w5609) -> ("SOH过低"=w5608:dbl)
                    n2184 = call "输入分辨率计算-EV05.vi"("1字节?"=FALSE, "数值"=w5608, "偏移量"=0.0, "分辨率"=0.1) -> ("低字节"=w5610:dbl, "高字节1"=w5611:dbl)  [unwired: 1 in, 5 out]
                    n2185 = call "二进制解析-8.6.vi"("索引"=4, "数值"=w5611) -> ("低位子数组"=w5614:i32[])  [unwired: 3 out]
                    n2186 = call "二进制解析-8.6.vi"("索引"=4, "数值"=w5610) -> ("低位子数组"=w5603:i32[], "高位子数组"=w5613:i32[])  [unwired: 2 out]
                    n2187 = call "二进制解析-8.6.vi"("索引"=4, "数值"=0) -> ("低位子数组"=w5604:i32[])  [unwired: 3 out]
                    n2188 = Insert Into Array(array=w5614, new element=w5613) -> (w5607:i32[])  [unwired: 1 in]
                    n2189 = Insert Into Array(array=w5603, new element=w5604) -> (w5602:i32[])  [unwired: 1 in]
                    n2190 = call "数值二进制转十进制-8.6.vi"("子数组"=w5607) -> ("十进制数值"=w5612:i32)  [unwired: 4 out]
                    n2191 = call "数值二进制转十进制-8.6.vi"("子数组"=w5602) -> ("十进制数值"=w5601:i32)  [unwired: 4 out]
                  }
                  frame Enabled {
                    w5620 = 255 ("高字节1")
                  }
                }
                n2192 = Build Array(w5599, w5597) -> (w5600:i32[])
              }
            }
            n2193 = Insert Into Array(array=w5406, new element=w5407) -> (w5405:dbl[])  [unwired: 1 in]
          }
          n2194 = Build Array(w5402) -> (w5401:dbl[][])
          n2195 = Build Array("二级故障阀值") -> (w5392:string[])
        }
        frame "整组电压不均衡(3)" {
          n2196 = Unbundle By Name(w5626) -> ("一级故障 3"=w5627:refnum<vi>)
          n2197 = property class="Clust (严格)"(reference=w5627) -> ("Value"=w5625:T4)  [unwired: 1 in, 2 out]
          n2198 = for {
            N: 17 -> [_]
            tunnel: w5625 -> [w5637]
            shift-right: [w5634] -> w5631
            shift-left: dbl[] [] -> [w5635]
            i -> [w5638]
            n2199 = case shown="13" w5638 {
              tunnel: w5637 -> [w5639 w5650 w5661 w5671 w5681 w5691 w5703 w5715 w5727 w5739 w5751 w5763 w5777 w5798 w5809 w5818 w5827]
              tunnel: [w5640 w5651 w5662 w5672 w5682 w5693 w5705 w5717 w5729 w5741 w5753 w5764 w5786 w5801 w5808 w5817 w5829] -> w5636
              frame 0, Default {
                # "总电压过高"
                n2200 = disable-structure shown="启用" {
                  disable-tunnel: [w5646 w5649] -> w5642
                  disable-tunnel: [w5645 w5649] -> w5641
                  disable-tunnel: w5639 -> [w5644 _]
                  frame Disabled {
                    n2201 = Unbundle By Name(w5644) -> ("总电压过高"=w5643:dbl)
                    n2202 = call "输入分辨率计算-EV05.vi"("1字节?"=FALSE, "数值"=w5643, "分辨率"=0.1) -> ("低字节"=w5646:dbl, "高字节1"=w5645:dbl)  [unwired: 2 in, 5 out]
                  }
                  frame Enabled {
                    w5649 = 255 ("高字节1")
                  }
                }
                n2203 = Build Array(w5641, w5642) -> (w5640:i32[])
              }
              frame 1 {
                # "总电压过低"
                n2204 = disable-structure shown="启用" {
                  disable-tunnel: [w5657 w5660] -> w5653
                  disable-tunnel: [w5656 w5660] -> w5652
                  disable-tunnel: w5650 -> [w5655 _]
                  frame Disabled {
                    n2205 = Unbundle By Name(w5655) -> ("总电压过低"=w5654:dbl)
                    n2206 = call "输入分辨率计算-EV05.vi"("1字节?"=FALSE, "数值"=w5654, "分辨率"=0.1) -> ("低字节"=w5657:dbl, "高字节1"=w5656:dbl)  [unwired: 2 in, 5 out]
                  }
                  frame Enabled {
                    w5660 = 255 ("高字节1")
                  }
                }
                n2207 = Build Array(w5652, w5653) -> (w5651:i32[])
              }
              frame 2 {
                # "温度过高"
                n2208 = disable-structure shown="启用" {
                  disable-tunnel: [w5667 255 ("高字节1")] -> w5663
                  disable-tunnel: w5661 -> [w5665 _]
                  frame Disabled {
                    n2209 = Unbundle By Name(w5665) -> ("温度过高"=w5664:dbl)
                    n2210 = call "输入分辨率计算-EV05.vi"("1字节?"=TRUE, "数值"=w5664, "偏移量"=-40.0, "分辨率"=1.0) -> ("高字节1"=w5667:dbl)  [unwired: 1 in, 6 out]
                  }
                  frame Enabled {
                  }
                }
                n2211 = Build Array(w5663) -> (w5662:i32[])
              }
              frame 3 {
                # "温度过低"
                n2212 = disable-structure shown="启用" {
                  disable-tunnel: [w5677 255 ("高字节1")] -> w5673
                  disable-tunnel: w5671 -> [w5675 _]
                  frame Disabled {
                    n2213 = Unbundle By Name(w5675) -> ("温度过低"=w5674:dbl)
                    n2214 = call "输入分辨率计算-EV05.vi"("1字节?"=TRUE, "数值"=w5674, "偏移量"=-40.0, "分辨率"=1.0) -> ("高字节1"=w5677:dbl)  [unwired: 1 in, 6 out]
                  }
                  frame Enabled {
                  }
                }
                n2215 = Build Array(w5673) -> (w5672:i32[])
              }
              frame 4 {
                # "整组温度不均衡"
                n2216 = disable-structure shown="启用" {
                  disable-tunnel: [w5687 255 ("高字节1")] -> w5683
                  disable-tunnel: w5681 -> [w5685 _]
                  frame Disabled {
                    n2217 = Unbundle By Name(w5685) -> ("整组温度不均衡"=w5684:dbl)
                    n2218 = call "输入分辨率计算-EV05.vi"("1字节?"=TRUE, "数值"=w5684, "偏移量"=0.0, "分辨率"=1.0) -> ("高字节1"=w5687:dbl)  [unwired: 1 in, 6 out]
                  }
                  frame Enabled {
                  }
                }
                n2219 = Build Array(w5683) -> (w5682:i32[])
              }
              frame 5 {
                # "单组电压不均衡"
                n2220 = disable-structure shown="启用" {
                  disable-tunnel: [w5699 w5702] -> w5694
                  disable-tunnel: [w5697 w5702] -> w5692
                  disable-tunnel: w5691 -> [w5696 _]
                  frame Disabled {
                    n2221 = Unbundle By Name(w5696) -> ("单组电压不均衡"=w5695:dbl)
                    n2222 = call "输入分辨率计算-EV05.vi"("1字节?"=FALSE, "数值"=w5695, "偏移量"=0.0, "分辨率"=0.001) -> ("低字节"=w5697:dbl, "高字节1"=w5699:dbl)  [unwired: 1 in, 5 out]
                  }
                  frame Enabled {
                    w5702 = 255 ("高字节1")
                  }
                }
                n2223 = Build Array(w5694, w5692) -> (w5693:i32[])
              }
              frame 6 {
                # "整组电压不均衡"
                n2224 = disable-structure shown="启用" {
                  disable-tunnel: [w5711 w5714] -> w5706
                  disable-tunnel: [w5709 w5714] -> w5704
                  disable-tunnel: w5703 -> [w5708 _]
                  frame Enabled {
                    n2225 = Unbundle By Name(w5708) -> ("整组电压不均衡"=w5707:dbl)
                    n2226 = call "输入分辨率计算-EV05.vi"("1字节?"=FALSE, "数值"=w5707, "偏移量"=0.0, "分辨率"=0.001) -> ("低字节"=w5709:dbl, "高字节1"=w5711:dbl)  [unwired: 1 in, 5 out]
                  }
                  frame Disabled {
                    w5714 = 255 ("高字节1")
                  }
                }
                n2227 = Build Array(w5706, w5704) -> (w5705:dbl[])
              }
              frame 7 {
                # "单体电压过高"
                n2228 = disable-structure shown="启用" {
                  disable-tunnel: [w5723 w5726] -> w5718
                  disable-tunnel: [w5721 w5726] -> w5716
                  disable-tunnel: w5715 -> [w5720 _]
                  frame Disabled {
                    n2229 = Unbundle By Name(w5720) -> ("单体电压过高"=w5719:dbl)
                    n2230 = call "输入分辨率计算-EV05.vi"("1字节?"=FALSE, "数值"=w5719, "偏移量"=0.0, "分辨率"=0.001) -> ("低字节"=w5721:dbl, "高字节1"=w5723:dbl)  [unwired: 1 in, 5 out]
                  }
                  frame Enabled {
                    w5726 = 255 ("高字节1")
                  }
                }
                n2231 = Build Array(w5718, w5716) -> (w5717:i32[])
              }
              frame 8 {
                # "单体电压过低"
                n2232 = disable-structure shown="启用" {
                  disable-tunnel: [w5735 w5738] -> w5730
                  disable-tunnel: [w5733 w5738] -> w5728
                  disable-tunnel: w5727 -> [w5732 _]
                  frame Disabled {
                    n2233 = Unbundle By Name(w5732) -> ("单体电压过低"=w5731:dbl)
                    n2234 = call "输入分辨率计算-EV05.vi"("1字节?"=FALSE, "数值"=w5731, "偏移量"=0.0, "分辨率"=0.001) -> ("低字节"=w5733:dbl, "高字节1"=w5735:dbl)  [unwired: 1 in, 5 out]
                  }
                  frame Enabled {
                    w5738 = 255 ("高字节1")
                  }
                }
                n2235 = Build Array(w5730, w5728) -> (w5729:i32[])
              }
              frame 9 {
                # "充电电流过高"
                n2236 = disable-structure shown="启用" {
                  disable-tunnel: [w5747 w5750] -> w5742
                  disable-tunnel: [w5745 w5750] -> w5740
                  disable-tunnel: w5739 -> [w5744 _]
                  frame Disabled {
                    n2237 = Unbundle By Name(w5744) -> ("充电电流过高"=w5743:dbl)
                    n2238 = call "输入分辨率计算-EV05.vi"("1字节?"=FALSE, "数值"=w5743, "偏移量"=-3000.0, "分辨率"=0.1) -> ("低字节"=w5745:dbl, "高字节1"=w5747:dbl)  [unwired: 1 in, 5 out]
                  }
                  frame Enabled {
                    w5750 = 255 ("高字节1")
                  }
                }
                n2239 = Build Array(w5742, w5740) -> (w5741:i32[])
              }
              frame 10 {
                # "放电电流过高"
                n2240 = disable-structure shown="启用" {
                  disable-tunnel: [w5759 w5762] -> w5754
                  disable-tunnel: [w5757 w5762] -> w5752
                  disable-tunnel: w5751 -> [w5756 _]
                  frame Disabled {
                    n2241 = Unbundle By Name(w5756) -> ("放电电流过高"=w5755:dbl)
                    n2242 = call "输入分辨率计算-EV05.vi"("1字节?"=FALSE, "数值"=w5755, "偏移量"=-3000.0, "分辨率"=0.1) -> ("低字节"=w5757:dbl, "高字节1"=w5759:dbl)  [unwired: 1 in, 5 out]
                  }
                  frame Enabled {
                    w5762 = 255 ("高字节1")
                  }
                }
                n2243 = Build Array(w5754, w5752) -> (w5753:i32[])
              }
              frame 11 {
                # "单组温度不均衡"
                n2244 = disable-structure shown="启用" {
                  disable-tunnel: [w5769 255 ("高字节1")] -> w5765
                  disable-tunnel: w5763 -> [w5767 _]
                  frame Disabled {
                    n2245 = Unbundle By Name(w5767) -> ("单组温度不均衡"=w5766:dbl)
                    n2246 = call "输入分辨率计算-EV05.vi"("1字节?"=TRUE, "数值"=w5766, "偏移量"=0.0, "分辨率"=1.0) -> ("高字节1"=w5769:dbl)  [unwired: 1 in, 6 out]
                  }
                  frame Enabled {
                  }
                }
                n2247 = Build Array(w5765) -> (w5764:i32[])
              }
              frame 12 {
                # "SOC过高"
                n2248 = Unbundle By Name(w5777) -> ("SOC过高"=w5776:dbl)
                n2249 = call "输入分辨率计算-EV05.vi"("1字节?"=FALSE, "数值"=w5776, "偏移量"=0.0, "分辨率"=0.1) -> ("低字节"=w5778:dbl, "高字节1"=w5779:dbl)  [unwired: 1 in, 5 out]
                n2250 = call "二进制解析-8.6.vi"("索引"=4, "数值"=w5779) -> ("低位子数组"=w5782:i32[])  [unwired: 3 out]
                n2251 = call "二进制解析-8.6.vi"("索引"=4, "数值"=w5778) -> ("低位子数组"=w5774:i32[], "高位子数组"=w5781:i32[])  [unwired: 2 out]
                n2252 = Insert Into Array(array=w5782, new element=w5781) -> (w5780:i32[])  [unwired: 1 in]
                n2253 = call "数值二进制转十进制-8.6.vi"("子数组"=w5780) -> ("十进制数值"=w5775:i32)  [unwired: 4 out]
                n2254 = disable-structure shown="启用" {
                  disable-tunnel: w5775 -> [w5790 _]
                  disable-tunnel: [w5790 255 ("高字节1")] -> w5773
                  disable-tunnel: [w5789 i32[] [] ("低位子数组 24")] -> _
                  disable-tunnel: w5774 -> [w5789 _]
                  frame Disabled {
                  }
                  frame Enabled {
                  }
                }
                n2255 = Build Array(w5773, w5773) -> (w5786:i32[])
              }
              frame 13 {
                # "SOC过低"
                n2256 = Unbundle By Name(w5798) -> ("SOC过低"=w5797:dbl)
                n2257 = call "输入分辨率计算-EV05.vi"("1字节?"=FALSE, "数值"=w5797, "偏移量"=0.0, "分辨率"=0.1) -> ("低字节"=w5795:dbl, "高字节1"=w5796:dbl)  [unwired: 1 in, 5 out]
